vi "Read object configuration.vi"(6 "Object name":string, 7 "Present":bool, 8 "Error In":errorcluster, 9 "type":variant, 10 "File path":path, 11 "object":refnum<class>) -> (0 "Error Out":errorcluster, 1 "Configuration":variant, 2 "File path out":path, 4 "Section out":string, 5 "found?":bool)   [LabVIEW 2019]
uses:
  <vilib>/Utility/config.llb/NI_LVConfig.lvlib
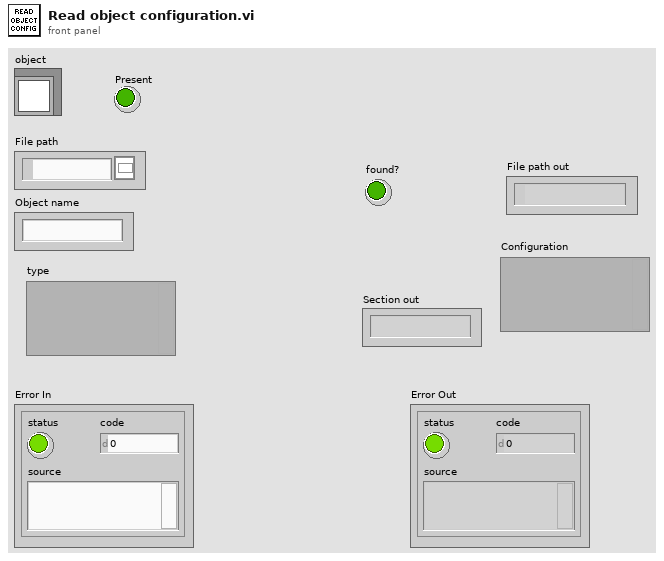
[diagram p1: front panel]
types:
  T1 = typedef "NI_LVConfig.lvlib/Config Data RefNum.ctl" = refnum<k1>
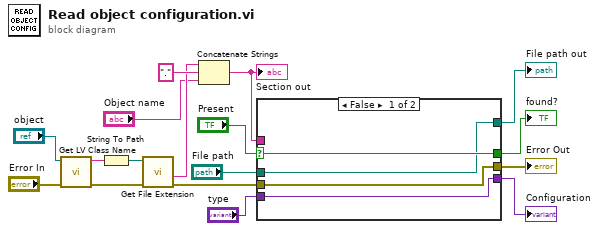
[diagram p0: block diagram]
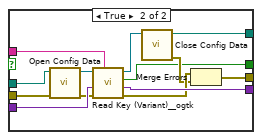
[diagram p2: hidden frame]
diagram:
  n1 = call <vilib>:"Get LV Class Name.vi"("error in (no error)"="Error In", "object"="object") -> ("error out"=w14:errorcluster, "class name"=w16:string)  [unwired: 8 in]
  n2 = String To Path(string=w16) -> (path=w12:path)
  n3 = call <vilib>:"Get File Extension.vi"("error in (no error)"=w14, "file"=w12) -> ("error out"=w15:errorcluster, "filename without extension"=w13:string)  [unwired: 5 in, 3 out]
  n4 = Concatenate Strings(w13, "." ("string"), "Object name") -> (w3:string)
  "Section out" <- w3
  n5 = case shown="False" "Present" {
    selector: "Present" -> [w20 _]
    tunnel: w15 -> [w19 w34]
    tunnel: "File path" -> [w18 w33]
    tunnel: "type" -> [w21 w32]
    tunnel: [w21 w31] -> w8
    tunnel: [w18 w25] -> w6
    tunnel: [w19 w24] -> w4
    tunnel: w3 -> [_ w23]
    tunnel: [w20 w22] -> w2
    frame False {
    }
    frame True {
      n6 = call <vilib>:"Open Config Data.vi"("error in (no error)"=w34, "configuration file path"=w33) -> ("error out"=w29:errorcluster, "refnum"=w30:T1)  [unwired: 7 in, 1 out]
      n7 = call <userlib>:"Read Key (Variant)__ogtk.vi"("section"=w23, "error in (no error)"=w29, "type"=w32, "refnum"=w30) -> ("error out"=w27:errorcluster, "key-value"=w31:variant, "found?"=w22:bool, "refnum out"=w28:T1)  [unwired: 4 in]
      n8 = call <vilib>:"Close Config Data.vi"("refnum"=w28) -> ("error out"=w26:errorcluster, "file path"=w25:path)  [unwired: 9 in]
      n9 = Merge Errors(w27, w26) -> (w24:errorcluster)
    }
  }
  "Configuration" <- w8
  "File path out" <- w6
  "Error Out" <- w4
  "found?" <- w2
